vi "Mallet Move Sensing Force SubVI.vi"(8 "Forward Speed":dbl, 9 "Reverse Speed":dbl, 10 "Forward Time":dbl=0.95 format="%#_13g", 11 "Reverse Time":dbl=0.95 format="%#_13g") -> (1 "Array of Forces":dbl[](array[numeric]), 2 "Average Force":dbl(graph))   [LabVIEW 2013]
doc: "An example that reads a user selectable analog input pin on the Arduino."
uses:
  <vilib>/LabVIEW Interface for Arduino/Type Defs/Pin Mode.ctl
  <vilib>/Analysis/baseanly.llb/Mean (DBL).vi
  <vilib>/LabVIEW Interface for Arduino/LabVIEW Interface for Arduino.lvlib
  <vilib>/Analysis/NI_AALBase.lvlib
panel:
  out "Elapsed Time (s)":dbl
  out "Average Force":dbl
  out "Force2 Average":dbl format="%0.2f"
  out "Force1 Average":dbl format="%0.2f"
  out "Force 2":dbl(graph)
  out "Voltage2":dbl(graph)
  out "Force":dbl(graph)
  out "Volatge":dbl(graph)
  out "Forard Duty Cycle":dbl
  out "Reverse Duty Cycle":dbl
  in  "stop 2":bool
  in  "stop":bool
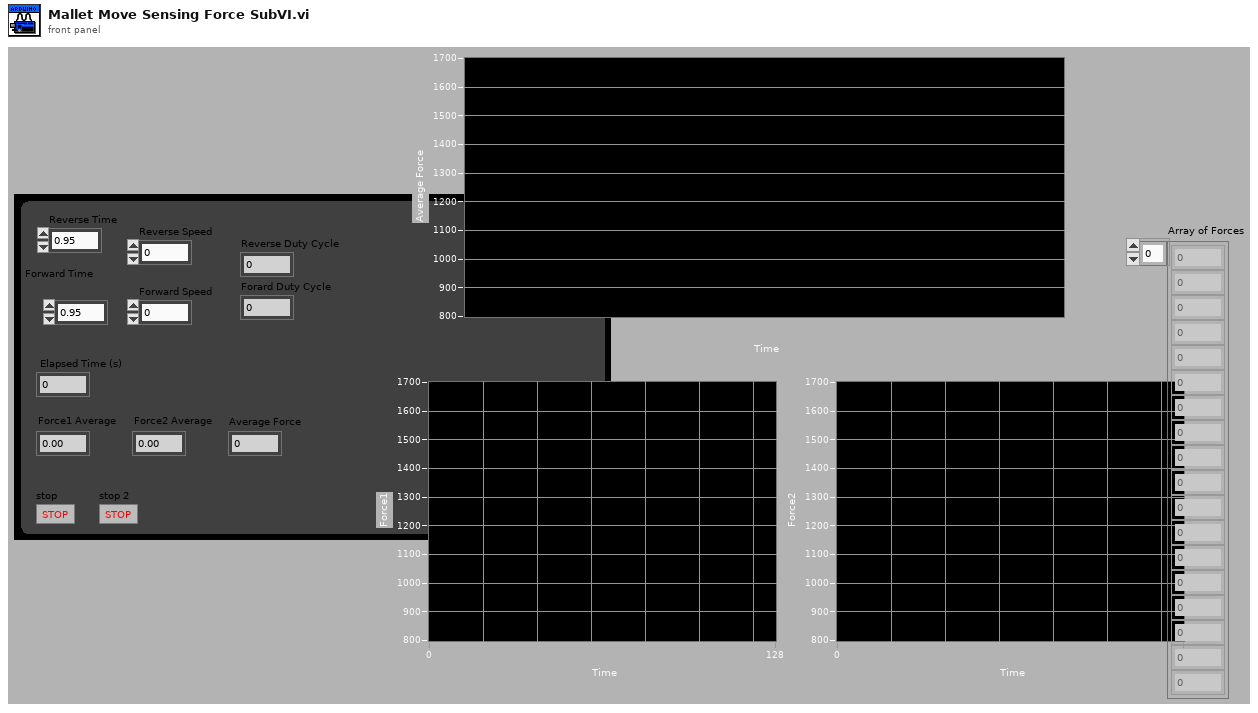
[diagram p1: front panel]
types:
  T1 = typedef "LabVIEW Interface for Arduino.lvlib/Pin Mode.ctl" = enum8{"Input", "Output"}
  T2 = typedef "LabVIEW Interface for Arduino.lvlib/Arduino Resource.ctl" = cluster{"VISA resource":refnum<visa-resource-name>, "Board Type":T3, "Connection Type":enum8{"USB / Serial"}, "Bytes Per Packet (15)":u8}
  T3 = typedef "LabVIEW Interface for Arduino.lvlib/Board Type.ctl" = enum16{"Uno", "Dimuelanove w/Atmega 328", "Mega 2560"}
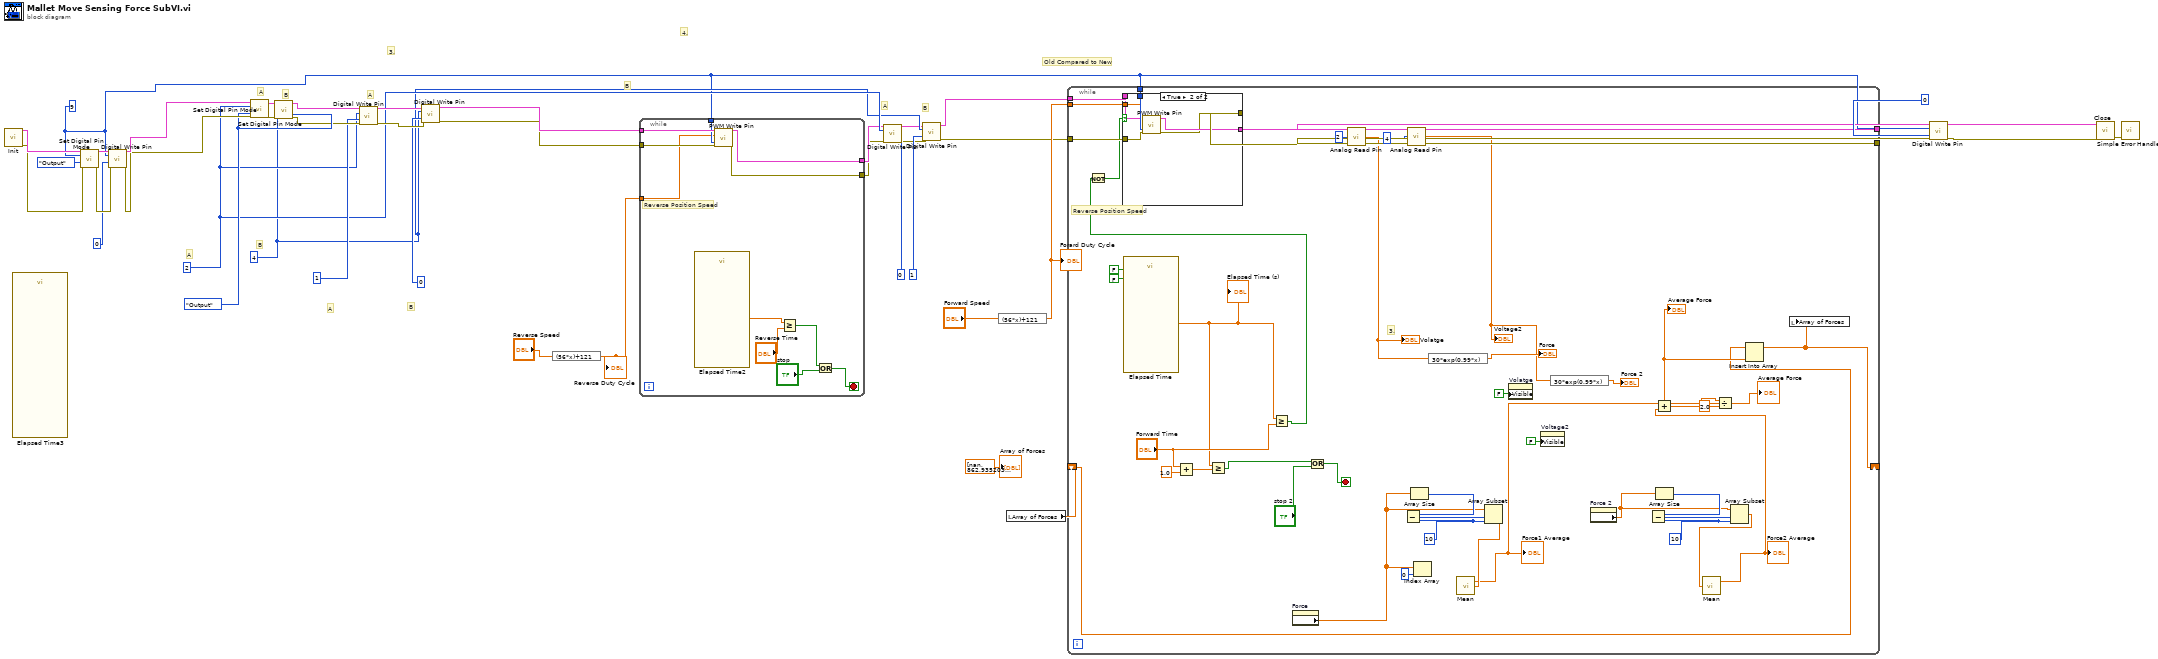
[diagram p0: block diagram]
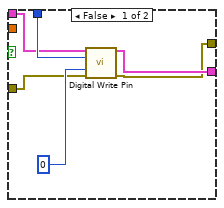
[diagram p2: hidden frame]
diagram:
  w9 = u8 9 ("PWM1 Pin")
  w16 = u8 4 ("Digital I/O Pin")
  w17 = u8 2 ("Digital I/O Pin")
  w30 = Pin_Mode."Output" ("Pin Mode (Input)")
  # "B"
  # "A"
  # "Old Compared to New"
  # "4."
  # "3."
  # "B"
  # "A"
  # "B"
  # "A"
  # "B"
  # "A"
  # "B"
  # "A"
  n1 = call <vilib>:"Init.vi"() -> ("Arduino Resource"=w34:T2, "error out"=w33:errorcluster)  [unwired: 18 in]
  n2 = call "Elapsed Time3"() -> ()  [unwired: 12 in, 8 out]
  n3 = call <vilib>:"Set Digital Pin Mode.vi"("Arduino Resource"=w34, "Digital I/O Pin"=w9, "Pin Mode (Input)"=Pin_Mode."Output", "error in"=w33) -> ("Arduino Resource"=w39:T2, "error out"=w38:errorcluster)  [unwired: 10 in]
  n4 = call <vilib>:"Digital Write Pin.vi"("Arduino Resource"=w39, "Digital I/O Pin (0)"=w9, "Value (0)"=u8 0, "error in"=w38) -> ("Arduino Resource"=w36:T2, "error out"=w35:errorcluster)  [unwired: 10 in]
  n5 = call <vilib>:"Set Digital Pin Mode.vi"("Arduino Resource"=w36, "Digital I/O Pin"=w17, "Pin Mode (Input)"=w30, "error in"=w35) -> ("Arduino Resource"=w29:T2, "error out"=w28:errorcluster)  [unwired: 10 in]
  n6 = call <vilib>:"Set Digital Pin Mode.vi"("Arduino Resource"=w29, "Digital I/O Pin"=w16, "Pin Mode (Input)"=w30, "error in"=w28) -> ("Arduino Resource"=w25:T2, "error out"=w24:errorcluster)  [unwired: 10 in]
  n7 = call <vilib>:"Digital Write Pin.vi"("Arduino Resource"=w25, "Digital I/O Pin (0)"=w17, "Value (0)"=u8 1 ("Reverse"), "error in"=w24) -> ("Arduino Resource"=w27:T2, "error out"=w26:errorcluster)  [unwired: 10 in]
  n8 = call <vilib>:"Digital Write Pin.vi"("Arduino Resource"=w27, "Digital I/O Pin (0)"=w16, "Value (0)"=u8 0 ("Forward"), "error in"=w26) -> ("Arduino Resource"=w21:T2, "error out"=w20:errorcluster)  [unwired: 10 in]
  n9 = expression code="(56*x)+121"("Reverse Speed") -> (w5:dbl)
  "Reverse Duty Cycle" <- w5
  n10 = while {
    tunnel: w21 -> [w53]
    tunnel: w20 -> [w52]
    tunnel: w9 -> [w51]
    tunnel: [w50] -> w15
    tunnel: [w49] -> w13
    tunnel: w5 -> [w43]
    stop <- w44 stop-if-true
    # "Reverse Position Speed"
    n11 = call "Elapsed Time2"() -> ("Elapsed Time (s)"=w47:dbl)  [unwired: 12 in, 7 out]
    n12 = call <vilib>:"PWM Write Pin.vi"("Arduino Resource"=w53, "Duty Cycle (0 - 255)"=w43, "PWM Pin (3)"=w51, "error in"=w52) -> ("Arduino Resource"=w50:T2, "error out"=w49:errorcluster)  [unwired: 10 in]
    n13 = Greater Or Equal?(x=w47, y="Reverse Time") -> (x >= y?=w46:bool)
    n14 = Or(x=w46, y="stop") -> (x .or. y?=w44:bool)
  }
  n15 = call <vilib>:"Digital Write Pin.vi"("Arduino Resource"=w15, "Digital I/O Pin (0)"=w17, "Value (0)"=u8 0 ("Reverse 2"), "error in"=w13) -> ("Arduino Resource"=w14:T2, "error out"=w12:errorcluster)  [unwired: 10 in]
  n16 = call <vilib>:"Digital Write Pin.vi"("Arduino Resource"=w14, "Digital I/O Pin (0)"=w16, "Value (0)"=u8 1 ("Forward 2"), "error in"=w12) -> ("Arduino Resource"=w4:T2, "error out"=w3:errorcluster)  [unwired: 10 in]
  n17 = expression code="(56*x)+121"("Forward Speed") -> (w7:dbl)
  "Forard Duty Cycle" <- w7
  n18 = local read "Array of Forces"() -> (w1:dbl[])
  n19 = while {
    tunnel: [w70] -> w11
    tunnel: [w69] -> w10
    tunnel: w9 -> [w98]
    tunnel: w7 -> [w97]
    tunnel: w4 -> [w96]
    tunnel: w3 -> [w95]
    shift-right: [w55] -> _
    shift-left: w1 -> [w54]
    stop <- w99 stop-if-true
    w82 = 10 ("length")
    w85 = 10 ("length")
    # "3."
    # "Reverse Position Speed"
    n20 = call "Elapsed Time"("Reset"=FALSE, "Auto Reset"=FALSE) -> ("Elapsed Time (s)"=w64:dbl)  [unwired: 10 in, 7 out]
    "Elapsed Time (s)" <- w64
    n21 = Add(x="Forward Time", y=1.0) -> (x+y=w65:dbl)
    n22 = Greater Or Equal?(x=w64, y=w65) -> (x >= y?=w63:bool)
    n23 = Greater Or Equal?(x=w64, y="Forward Time") -> (x >= y?=w61:bool)
    n24 = Not(x=w61) -> (.not. x?=w62:bool)
    n25 = case shown="True" w62 {
      tunnel: w98 -> [w106 w112]
      tunnel: w97 -> [_ w111]
      tunnel: w96 -> [w103 w110]
      tunnel: w95 -> [w104 w109]
      tunnel: [w102 w108] -> w72
      tunnel: [w101 w107] -> w71
      frame False {
        n26 = call <vilib>:"Digital Write Pin.vi"("Arduino Resource"=w103, "Digital I/O Pin (0)"=w106, "Value (0)"=u8 0, "error in"=w104) -> ("Arduino Resource"=w102:T2, "error out"=w101:errorcluster)  [unwired: 10 in]
      }
      frame True {
        n27 = call <vilib>:"PWM Write Pin.vi"("Arduino Resource"=w110, "Duty Cycle (0 - 255)"=w111, "PWM Pin (3)"=w112, "error in"=w109) -> ("Arduino Resource"=w108:T2, "error out"=w107:errorcluster)  [unwired: 10 in]
      }
    }
    n28 = property on="Force" class="WFChart (strict)"() -> ("History Data"=w58:dbl[])  [unwired: 2 in, 2 out]
    n29 = Or(x=w63, y="stop 2") -> (x .or. y?=w99:bool)
    n30 = call <vilib>:"Analog Read Pin.vi"("Arduino Resource"=w72, "Analog Input Pin (0)"=u8 2, "error in"=w71) -> ("Arduino Resource"=w91:T2, "Voltage"=w73:dbl, "error out"=w90:errorcluster)  [unwired: 10 in]
    "Volatge" <- w73
    n31 = call <vilib>:"Analog Read Pin.vi"("Arduino Resource"=w91, "Analog Input Pin (0)"=u8 4, "error in"=w90) -> ("Arduino Resource"=w70:T2, "Voltage"=w89:dbl, "error out"=w69:errorcluster)  [unwired: 10 in]
    "Voltage2" <- w89
    n32 = Array Size(array=w58) -> (size(s)=w86:i32)
    n33 = Subtract(x=w86, y=w85) -> (x-y=w84:i32)
    n34 = Index Array(array=w58, index=0) -> ()  [unwired: 1 out]
    n35 = expression code="30*exp(0.99*x)"(w73) -> (→"Force":dbl)
    n36 = Array Subset(array=w58, index=w84, length=w85) -> (w87:dbl[])
    n37 = call-poly <vilib>:"Mean.vi"("X"=w87) -> ("mean"=w77:dbl)  [unwired: 1 out]
    "Force1 Average" <- w77
    n38 = property on="Volatge" class="WFChart (strict)"("Visible"=FALSE) -> ()  [unwired: 2 in, 2 out]
    n39 = property on="Voltage2" class="WFChart (strict)"("Visible"=FALSE) -> ()  [unwired: 2 in, 2 out]
    n40 = expression code="30*exp(0.99*x)"(w89) -> (→"Force 2":dbl)
    n41 = property on="Force 2" class="WFChart (strict)"() -> ("History Data"=w80:dbl[])  [unwired: 2 in, 2 out]
    n42 = Array Size(array=w80) -> (size(s)=w83:i32)
    n43 = Subtract(x=w83, y=w82) -> (x-y=w81:i32)
    n44 = Array Subset(array=w80, index=w81, length=w82) -> (w79:dbl[])
    n45 = call-poly <vilib>:"Mean.vi"("X"=w79) -> ("mean"=w76:dbl)  [unwired: 1 out]
    "Force2 Average" <- w76
    n46 = Add(x=w77, y=w76) -> (x+y=w75:dbl)
    n47 = Divide(x=w75, y=2.0) -> (x/y=w56:dbl)
    "Average Force" <- w56
    "Average Force" <- w56
    n48 = Insert Into Array(array=w54, new element=w56) -> (w55:dbl[])  [unwired: 1 in]
    n49 = local write "Array of Forces"(w55) -> ()
  }
  n50 = call <vilib>:"Digital Write Pin.vi"("Arduino Resource"=w11, "Digital I/O Pin (0)"=w9, "Value (0)"=u8 0, "error in"=w10) -> ("Arduino Resource"=w41:T2, "error out"=w40:errorcluster)  [unwired: 10 in]
  n51 = call <vilib>:"Close.vi"("Arduino Resource"=w41, "error in"=w40) -> ("error out"=w42:errorcluster)  [unwired: 13 in]
  n52 = call <vilib>:"Simple Error Handler.vi"("error in (no error)"=w42) -> ()  [unwired: 4 in, 5 out]
  "Array of Forces" <- dbl[] [nan, 862.9352036334489, 861.7477905144149, 862.1435948874262, 862.3414970739318, 862.4602383858353, 862.5393992604374, 862.5959427422963, 862.3414970739318, 862.4074644694338, 862.4602383858353, 862.2227557620284, 862.4602383858353, 862.4602383858353, 862.4602383858353, 862.4602383858353, 862.4602383858353, 862.4602383858353, 862.697721009642, 862.697721009642, 862.4602383858353, 862.697721009642, 862.697721009642, 862.697721009642, 862.697721009642, 862.697721009642, 862.697721009642, 862.697721009642, 862.697721009642, 862.4602383858353, 862.697721009642, 862.697721009642, 862.4602383858353, 862.4602383858353, 862.2227557620284, 861.9852731382216, 861.9852731382216, 861.7477905144149, 861.7477905144149, 861.9852731382216, 861.9852731382216, 861.9852731382216, 862.2227557620284, 862.2227557620284, 862.2227557620284, 862.2227557620284, 861.9852731382216, 862.2227557620284, 862.2227557620284, 862.2227557620284, 862.2227557620284, 861.9852731382216, 861.9852731382216, 861.9852731382216, 862.2227557620284, 862.4602383858353, 862.4602383858353, 862.4602383858353, 862.2227557620284, 862.2227557620284, 862.2227557620284, 862.4602383858353, 862.4602383858353, 862.4602383858353, 862.4602383858353, 862.4602383858353, 862.697721009642, 862.697721009642, 862.9352036334489, 862.697721009642, 862.697721009642, 862.697721009642, 862.4602383858353, 862.4602383858353, 862.4602383858353, 862.4602383858353, 862.4602383858353, 862.4602383858353, 862.4602383858353, 862.697721009642, 862.4602383858353, 862.2227557620284, 862.4602383858353, 862.4602383858353, 862.4602383858353, 862.2227557620284, 862.2227557620284, 862.2227557620284, 862.2227557620284, 861.9852731382216, 862.2227557620284, 862.4602383858353, 862.4602383858353, 862.4602383858353, 862.4602383858353, 862.697721009642, 862.697721009642] ("Array of Forces")
